vi "post_pelletron.vi"(8 "error in (no error)":errorcluster, 11 "Pelletron Data":T1={"ID"=8, "Integer Timestamp"=2, "High Voltage"=3.0, "+ High Voltage Supply"=4.0, "- High Voltage Supply"=5.0, "HV Control Difference"=6.0, "Vacuum Pressure"=7.0, "Radiation"=8.0, "Column Current"=9.0, "Lost Charge"=54.0, "Chain Current"=3.0, "Control High Voltage"=0.0}) -> (0 "error out":errorcluster)   [LabVIEW 2013]
doc: "Adds a the given cluster to the pelletron_data table."
uses:
  User Interface/Controls/Pelletron.ctl
panel:
  # "Pelletron"
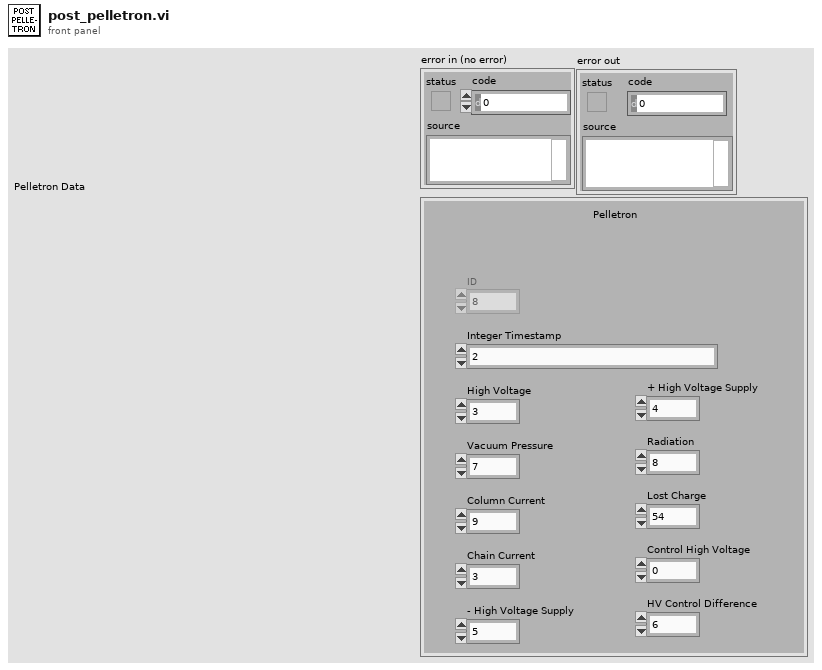
[diagram p1: front panel]
types:
  T1 = typedef "Pelletron.ctl" = cluster{"ID":i32, "Integer Timestamp":u64, "High Voltage":sgl, "+ High Voltage Supply":sgl, "- High Voltage Supply":sgl, "HV Control Difference":sgl, "Vacuum Pressure":sgl, "Radiation":sgl, "Column Current":sgl, "Lost Charge":sgl, "Chain Current":sgl, "Control High Voltage":sgl}
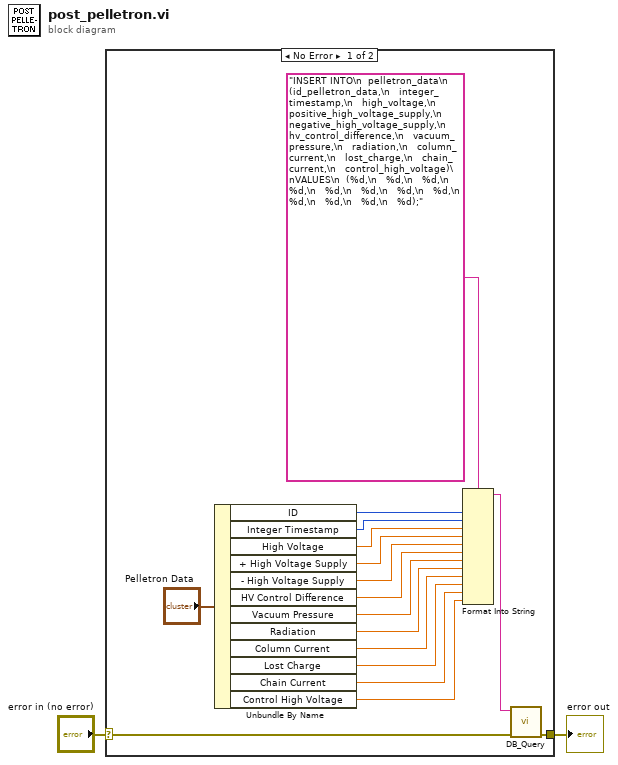
[diagram p0: block diagram]
diagram:
  n1 = case shown="No Error" "error in (no error)" {
    selector: "error in (no error)" -> [w5 w20]
    tunnel: [w3 w20] -> w1
    frame No Error {
      n2 = Unbundle By Name("Pelletron Data") -> ("ID"=w8:i32, "Integer Timestamp"=w9:u64, "High Voltage"=w10:sgl, "+ High Voltage Supply"=w11:sgl, "- High Voltage Supply"=w12:sgl, "HV Control Difference"=w13:sgl, "Vacuum Pressure"=w14:sgl, "Radiation"=w15:sgl, "Column Current"=w16:sgl, "Lost Charge"=w17:sgl, "Chain Current"=w18:sgl, "Control High Voltage"=w19:sgl)
      n3 = Format Into String(format string="INSERT INTO\n  pelletron_data\n  (id_pelletron_data,\n   integer_timestamp,\n   high_voltage,\n   positive_high_voltage_supply,\n   negative_high_voltage_supply,\n   hv_control_difference,\n   vacuum_pressure,\n   radiation,\n   column_current,\n   lost_charge,\n   chain_current,\n   control_high_voltage)\nVALUES\n  (%d,\n   %d,\n   %d,\n   %d,\n   %d,\n   %d,\n   %d,\n   %d,\n   %d,\n   %d,\n   %d,\n   %d);" ("Parameterized Query"), w8, w9, w10, w11, w12, w13, w14, w15, w16, w17, w18, w19) -> (resulting string=w4:string)  [unwired: 2 in, 1 out]
      n4 = call "DB_Query.vi"("error in (no error)"=w5, "Parameterized Query"=w4) -> ("error out"=w3:errorcluster)  [unwired: 7 in, 2 out]
    }
    frame Error {
    }
  }
  "error out" <- w1
